vi "Review Modules Dialog.vi"(8 "error in":errorcluster, 11 "Potting Procedure in":refnum<class "Potting Procedure.lvclass">) -> (0 "error out":errorcluster, 2 "Canceled":bool, 3 "Potting Procedure out":refnum<class "Potting Procedure.lvclass">)   [LabVIEW 2017]
uses:
  Shared Components/Vec3d Class/Vec3d Class.lvclass
  Shared Components/Utils/Type Definitions/Fiducial with Source.ctl
  <vilib>/vision/Image Controls.llb/IMAQ Image.ctl
  Shared Components/Utils/Type Definitions/Physical Image.ctl
  Shared Components/Utils/Type Definitions/Multi-Fiducial Image.ctl
  Shared Components/Utils/Type Definitions/Fiducial Image.ctl
  Procedure Classes/Potting Procedure/Type Definitions/Inspect Modules.ctl
  Procedure Classes/Potting Procedure/Type Definitions/Review Modules.ctl
  Procedure Classes/Potting Procedure/Type Definitions/Inspect Modules - Module.ctl
  Procedure Classes/Potting Procedure/Potting Procedure.lvclass
panel:
  out "Current Module":cluster{"Chuck":i32, "Slot":i32}={"Chuck"=1, "Slot"=1}
  out "idx_label":string="1/10"
  in  "idx":i32
  in  "Previous":bool
  in  "Next":bool
  in  "Tab Control":T1(tab)
  in  "HDI ROC 0":bool
  in  "HDI ROC 9":bool
  in  "HDI ROC 10":bool
  in  "HDI ROC 11":bool
  in  "HDI ROC 12":bool
  in  "HDI ROC 13":bool
  in  "HDI ROC 14":bool
  in  "HDI ROC 15":bool
  in  "HDI ROC 8":bool
  in  "HDI ROC 6":bool
  in  "HDI ROC 5":bool
  in  "HDI ROC 4":bool
  in  "HDI ROC 3":bool
  in  "HDI ROC 2":bool
  in  "HDI ROC 1":bool
  out "HDI BR":T2(plugin-control)
  out "HDI BL":T2(plugin-control)
  out "HDI TR":T2(plugin-control)
  out "HDI TL":T2(plugin-control)
  in  "HDI ROC 7":bool
  in  "BBM ROC 0":bool
  in  "BBM ROC 9":bool
  in  "BBM ROC 10":bool
  in  "BBM ROC 11":bool
  in  "BBM ROC 12":bool
  in  "BBM ROC 13":bool
  in  "BBM ROC 14":bool
  in  "BBM ROC 15":bool
  in  "BBM ROC 8":bool
  in  "BBM ROC 6":bool
  in  "BBM ROC 5":bool
  in  "BBM ROC 4":bool
  in  "BBM ROC 3":bool
  in  "BBM ROC 2":bool
  in  "BBM ROC 1":bool
  in  "BBM ROC 7":bool
  out "BBM TL":T2(plugin-control)
  out "BBM TR":T2(plugin-control)
  out "BBM BL":T2(plugin-control)
  out "BBM BR":T2(plugin-control)
  in  "TBM Inner Bottom":bool
  in  "TBM Outer Bottom":bool
  in  "TBM Outer Top":bool
  in  "TBM Outer Right":bool
  in  "TBM Outer Left":bool
  in  "TBM Inner Right":bool
  in  "TBM Inner Left":bool
  in  "TBM Inner Top":bool
  out "TBM-HDI":T2(plugin-control)
  out "TBM-TBM":T2(plugin-control)
  in  "High Voltage Sensor":bool
  in  "High Voltage HDI":bool
  in  "Address Pads Upper":bool
  in  "Address Pads Lower":bool
  out "addr":T2(plugin-control) caption="Address Pads"
  out "HV-HDI":T2(plugin-control)
  out "HV-BBM":T2(plugin-control)
  in  "OK Button":bool
  in  "Cancel Button":bool
  # "Click on images to correct reference positions.\nAll error fiducials must be corrected before continuing."
  # "Pattern Recognition"
  # "Error"
  # "User Defined"
  # "Default"
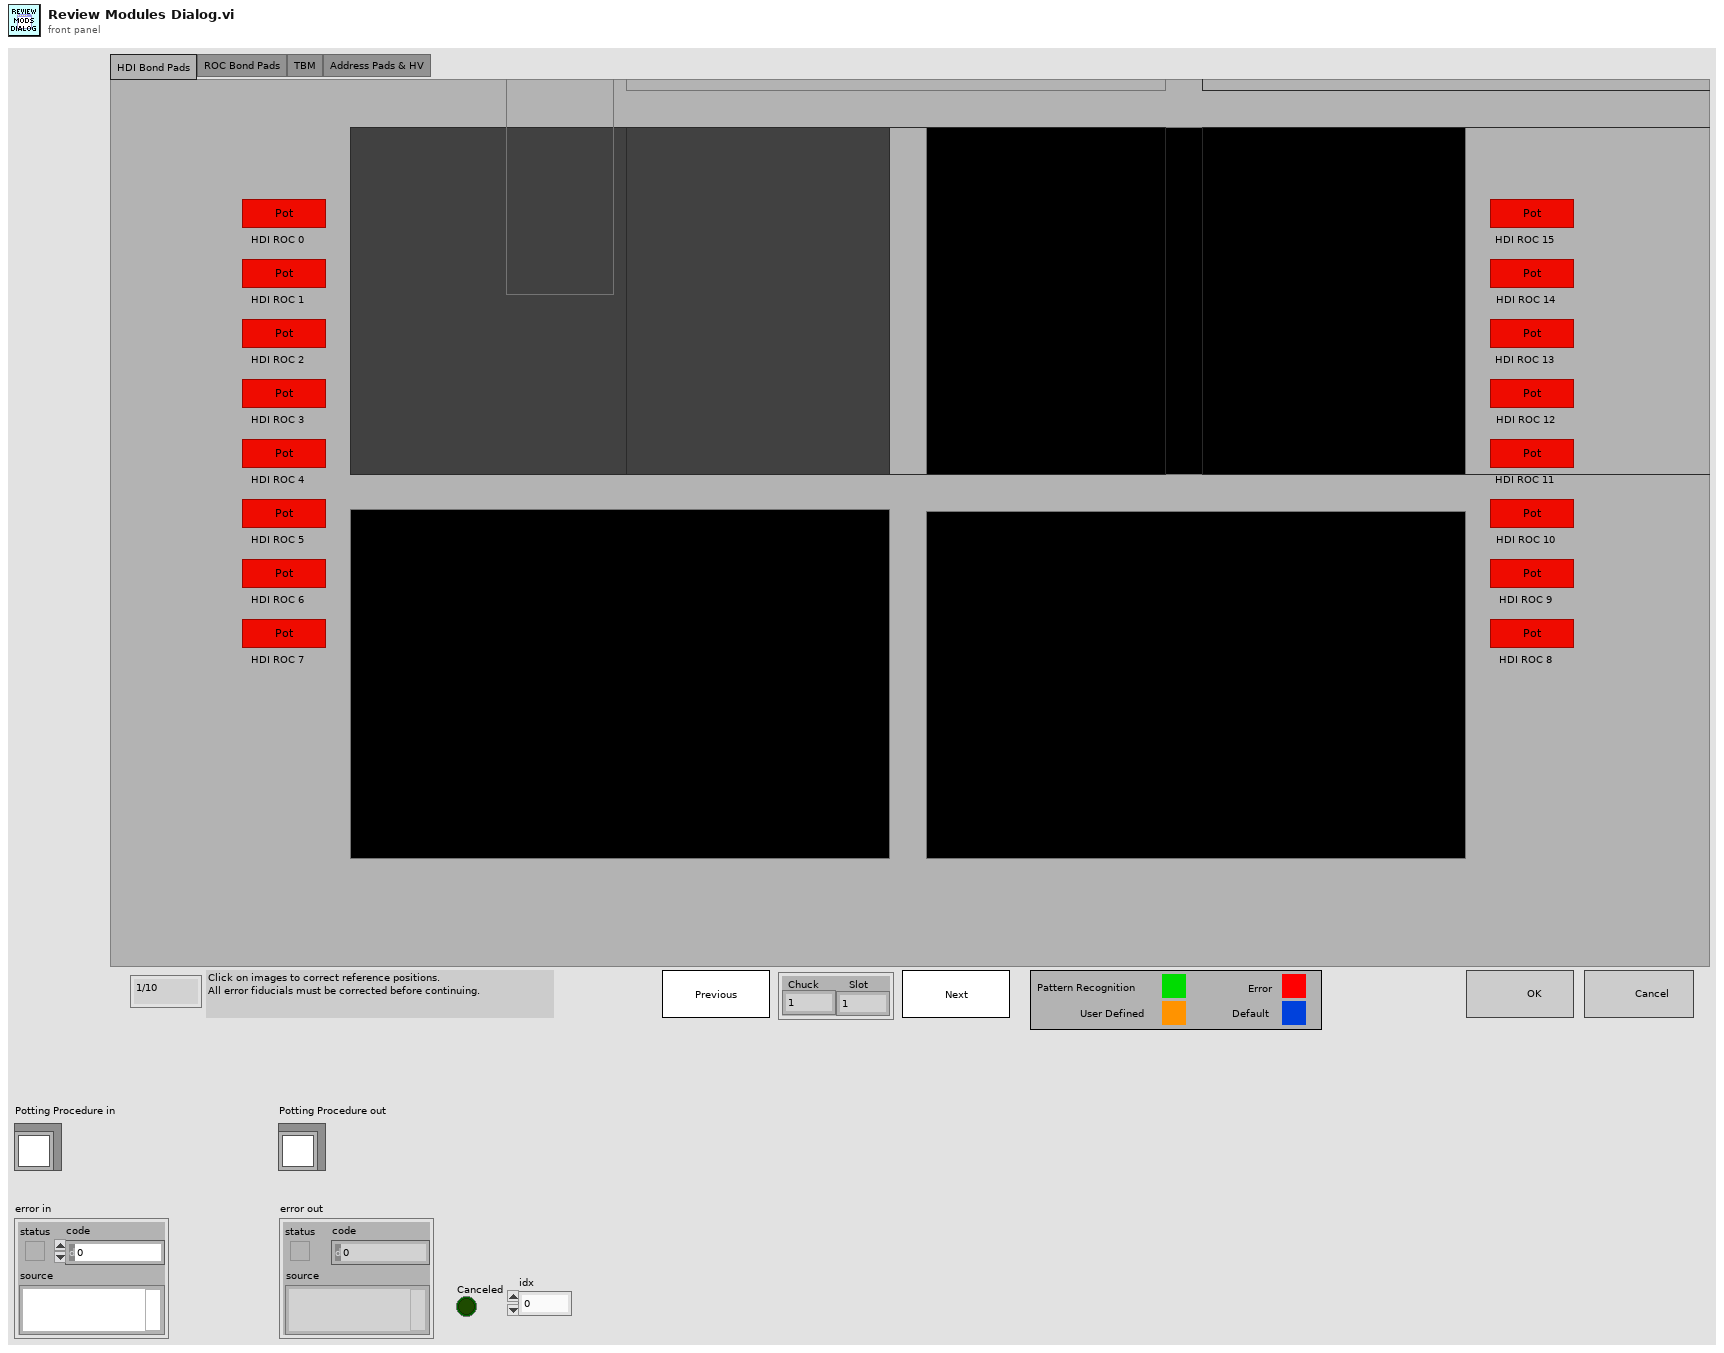
[diagram p1: front panel]
types:
  T1 = enum32{"HDI Bond Pads", "ROC Bond Pads", "TBM", "Address Pads & HV"}
  T2 = typedef "IMAQ Image.ctl" = refnum<image>
  T3 = cluster{"HDI Bond Pads":refnum<vi>[], "BBM Bond Pads":refnum<vi>[], "TBM Inner":refnum<vi>[], "TBM Outer":refnum<vi>[], "High Voltage":refnum<vi>[], "Address Pads":refnum<vi>[]}
  T4 = typedef "Inspect Modules.ctl" = cluster{"Has Been Run?":bool, "Module Positions":T5[]}
  T5 = typedef "Inspect Modules - Module.ctl" = cluster{"TBM-TBM":T6, "TBM-HDI":T6, "Address Pads":T6, "HDI Bond Pad References":T9[], "BBM Bond Pad References":T9[], "HV-HDI":T9, "HV-BBM":T9, "Chuck":i32, "Slot":i32, "Potting Selection":cluster{"HDI Bond Pads":bool[], "BBM Bond Pads":bool[], "TBM Inner":cluster{"Top":bool, "Left":bool, "Bottom":bool, "Right":bool}, "TBM Outer":cluster{"Top":bool, "Left":bool, "Bottom":bool, "Right":bool}, "Address Pads":cluster{"Top":bool, "Bottom":bool}, "High Voltage":cluster{"HDI":bool, "BBM":bool}}}
  T6 = typedef "Multi-Fiducial Image.ctl" = cluster{"Fiducial Image":T7, "Fiducials":cluster{"Selected Fiducial":T8, "fiducial name":string}[]}
  T7 = typedef "Physical Image.ctl" = cluster{"Image Position":refnum<class "Vec3d Class.lvclass">, "Image Reference":T2, "Field of View":cluster{"x(mm)":dbl, "y(mm)":dbl}}
  T8 = typedef "Fiducial with Source.ctl" = cluster{"Fiducial Image Coordinate":refnum<class "Vec3d Class.lvclass">, "Fiducial Source":enum16{"Pattern Recognition", "User", "Error", "Default"}}
  T9 = typedef "Fiducial Image.ctl" = cluster{"Fiducial Image":T7, "Selected Fiducial":T8, "fiducial name":string}
  T10 = enum16{"Pattern Recognition", "User", "Error", "Default"}
  T11 = cluster{"Top":bool, "Left":bool, "Bottom":bool, "Right":bool}
  T12 = typedef "LVPoint32TypeDef.ctl" = cluster{"Horizontal":i32, "Vertical":i32}
  T13 = cluster{"Selected Fiducial":T8, "fiducial name":string}[]
  T14 = cluster{"Selected Fiducial":T8, "fiducial name":string}
  T15 = cluster{"HDI Bond Pads":bool[], "BBM Bond Pads":bool[], "TBM Inner":cluster{"Top":bool, "Left":bool, "Bottom":bool, "Right":bool}, "TBM Outer":cluster{"Top":bool, "Left":bool, "Bottom":bool, "Right":bool}, "Address Pads":cluster{"Top":bool, "Bottom":bool}, "High Voltage":cluster{"HDI":bool, "BBM":bool}}
  T16 = typedef "eventvkey.ctl" = enum16{"ASCII", "Enter", "Return", "Shift", "Ctrl", "Alt", "Cmd", "Opt", "Caps", "NumLock", "Clear", "Break", "Up", "Down", "Left", "Right", "Insert", "Delete", "Home", "End", "PageUp", "PageDown", "Escape", "Help", "Pause", "ScrollLock", "F1", "F2", "F3", "F4", "F5", "F6", "F7", "F8", "F9", "F10", "F11", "F12", "F13", "F14", "F15", "F16", "F17", "F18", "F19", "F20", "F21", "F22", "F23", "F24", "Play", "VolumeUp", "VolumeDown", "Mute", "Two Byte Char"}
  T17 = typedef "Review Modules.ctl" = cluster{"Has Been Run?":bool}
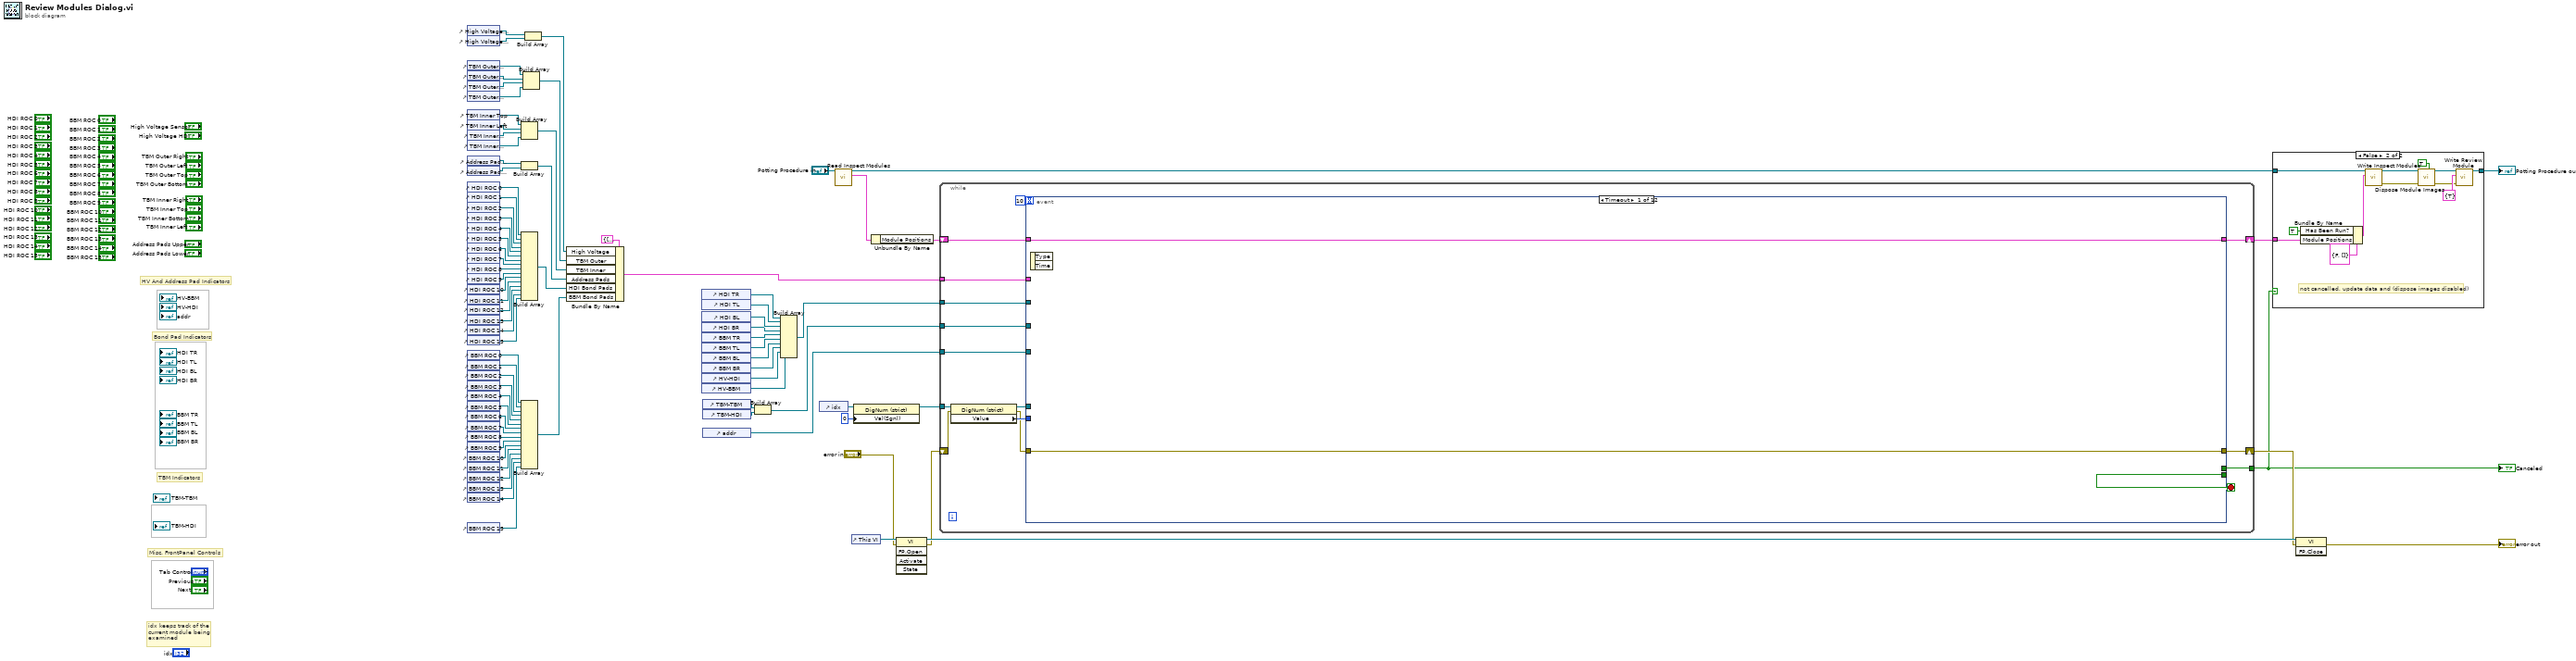
[diagram p0: block diagram]
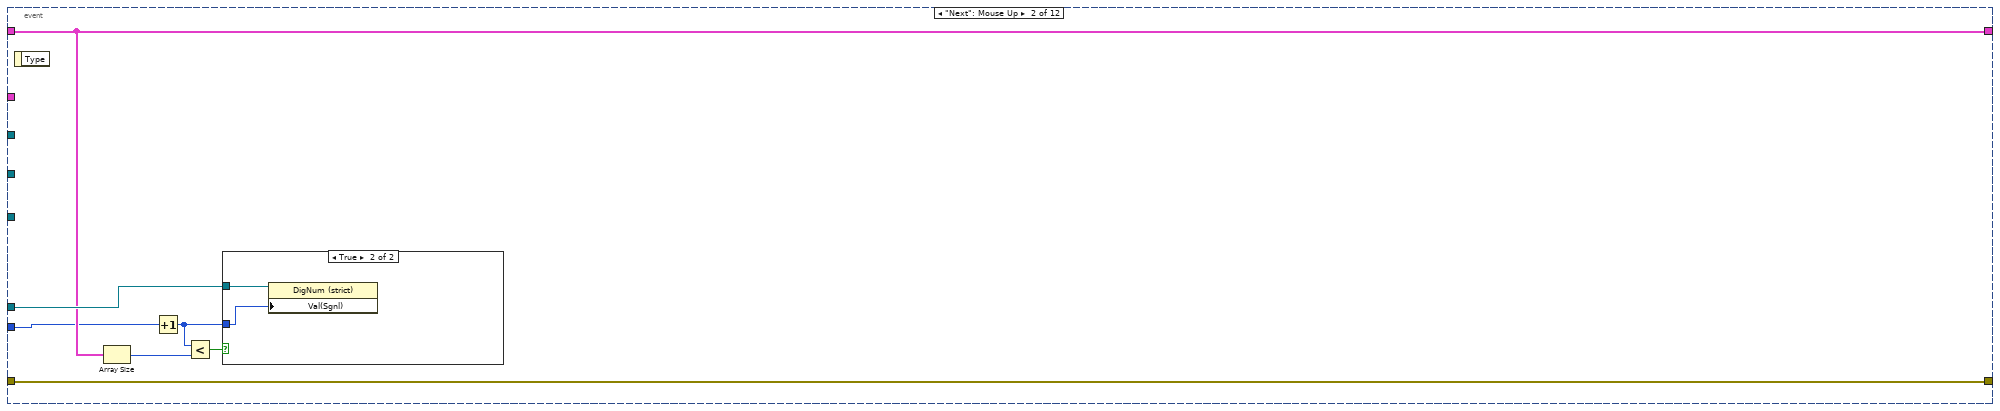
[diagram p3: hidden frame]
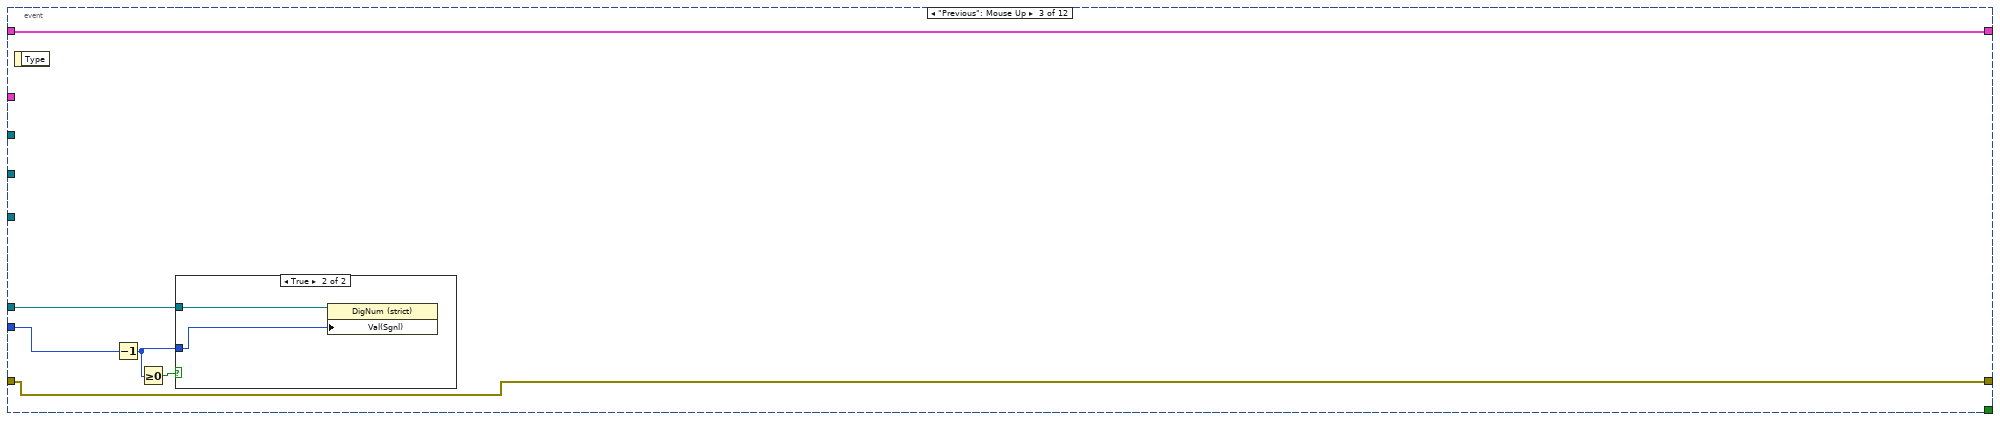
[diagram p5: hidden frame]
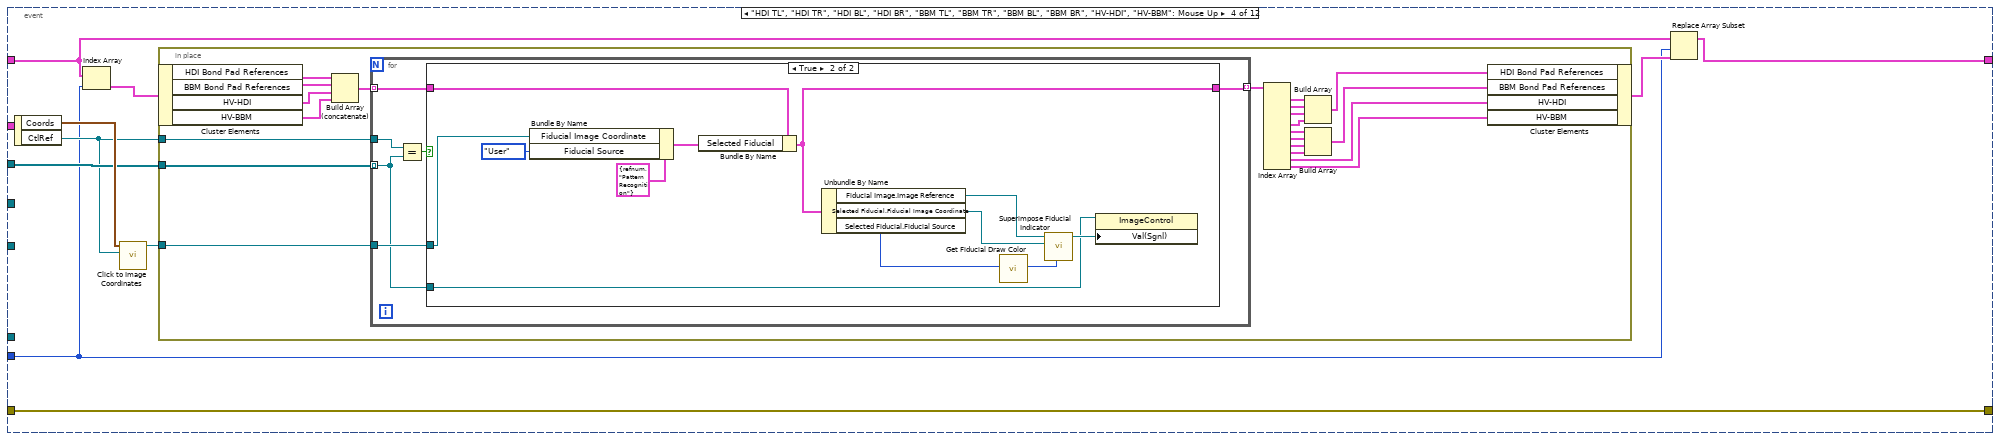
[diagram p7: hidden frame]
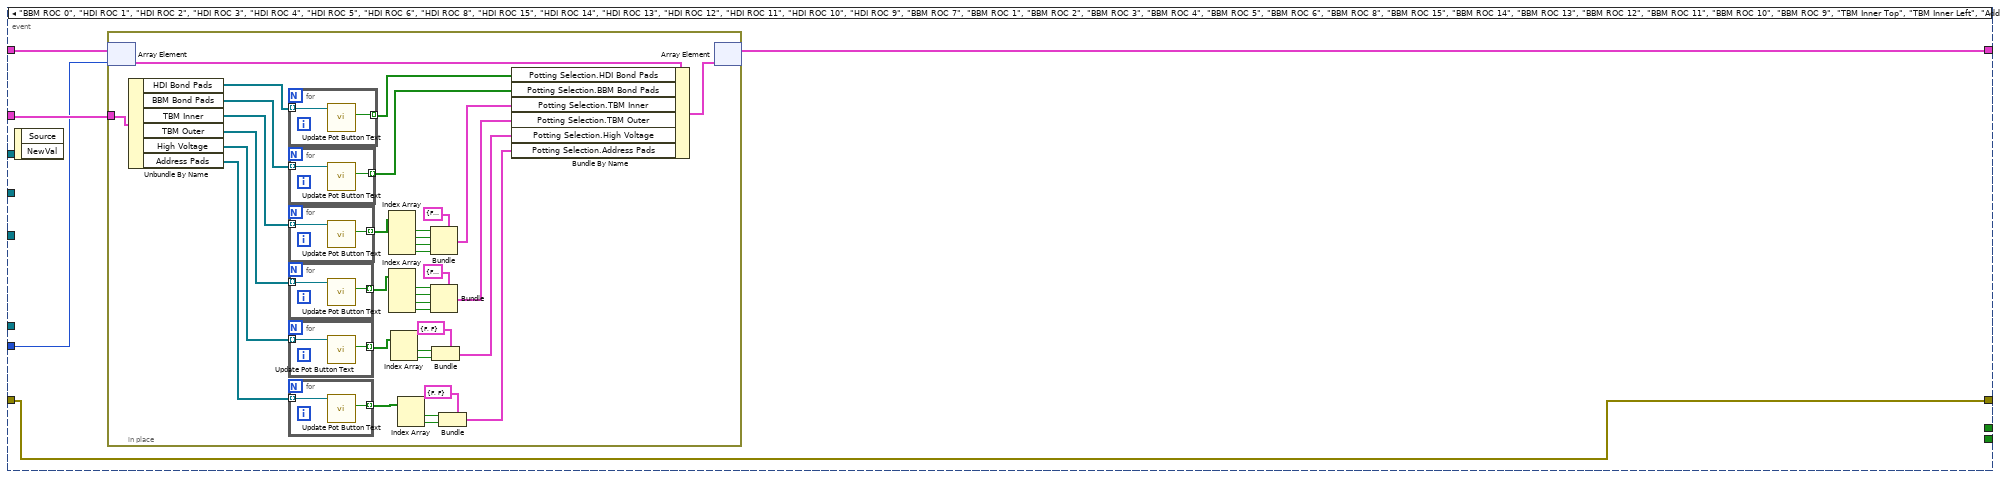
[diagram p9: hidden frame]
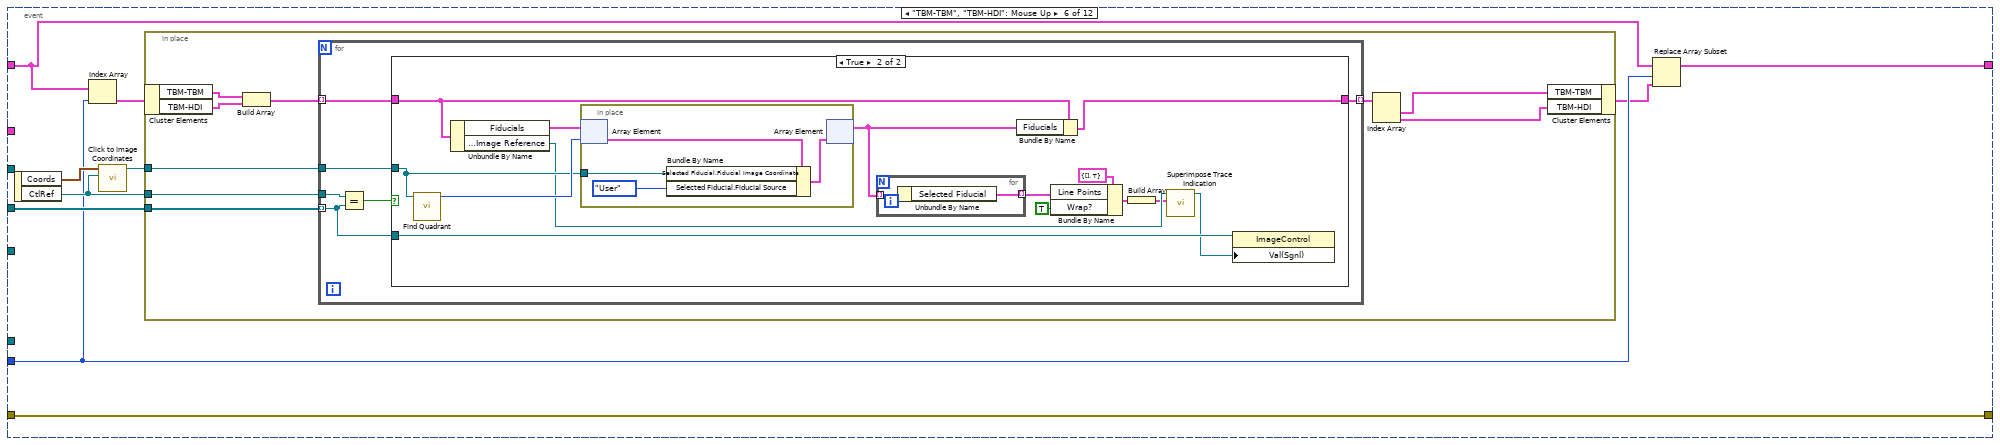
[diagram p10: hidden frame]
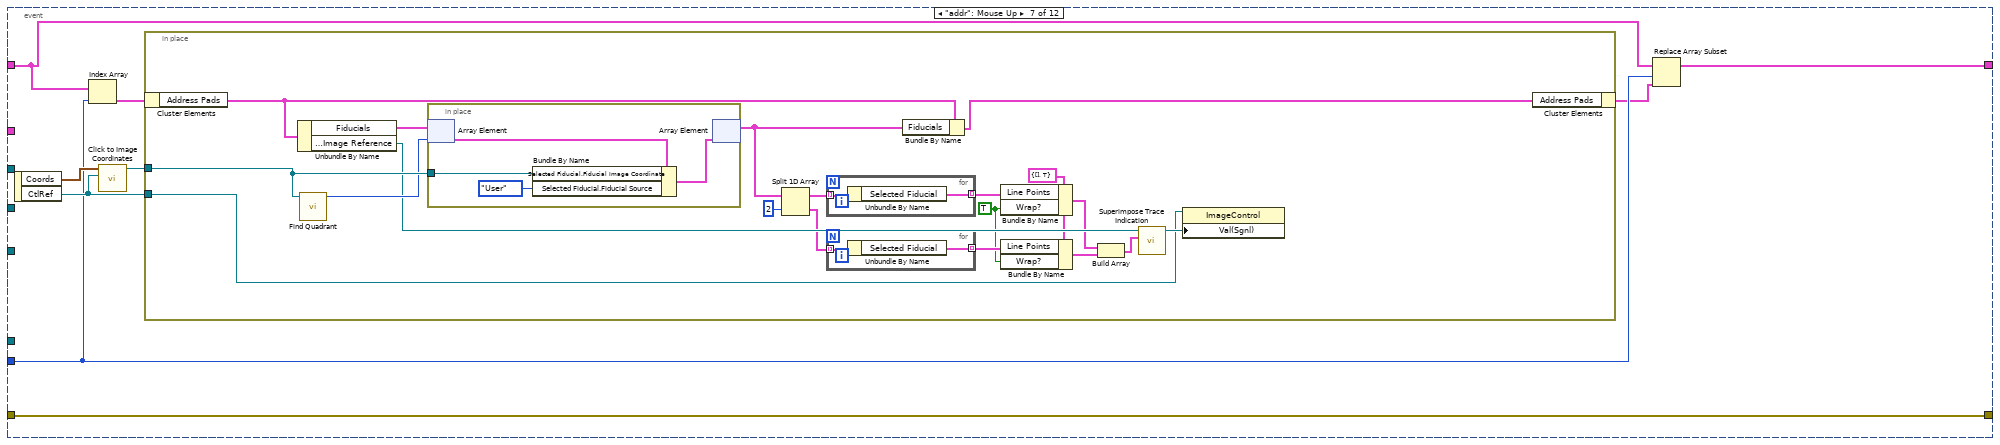
[diagram p12: hidden frame]
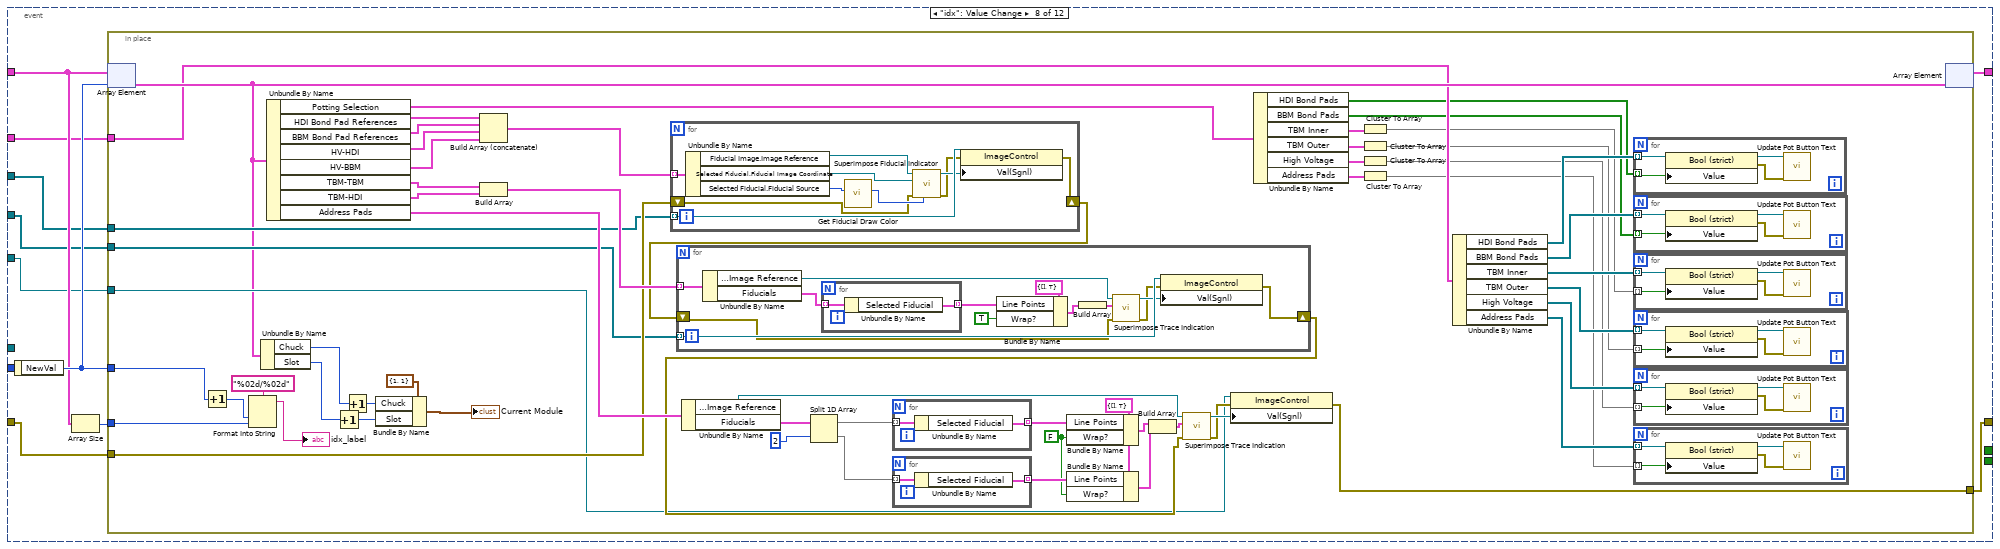
[diagram p13: hidden frame]
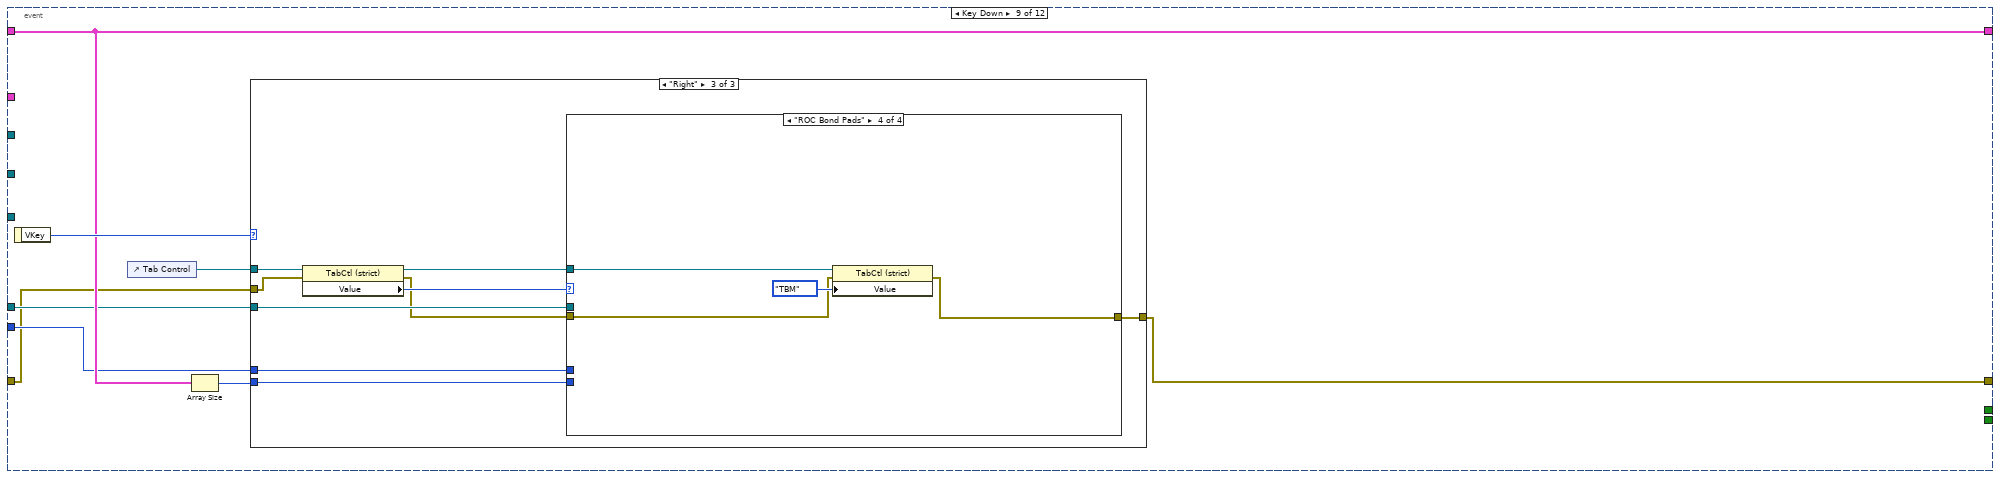
[diagram p14: hidden frame]
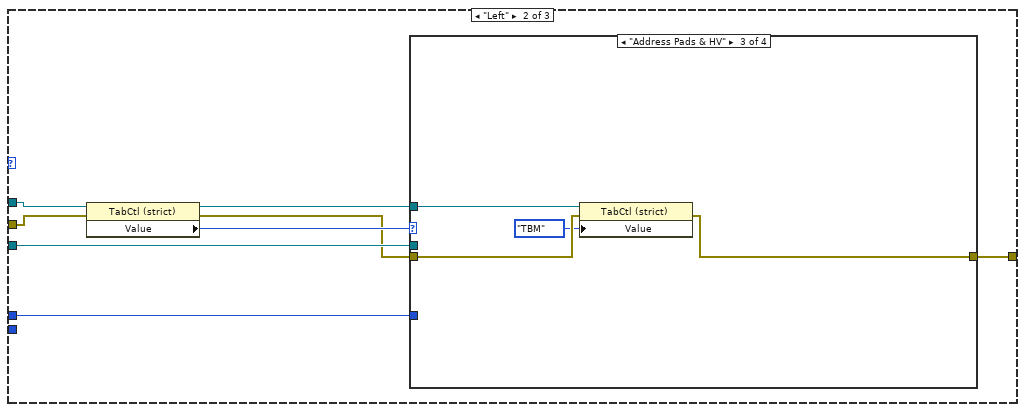
[diagram p16: hidden frame]
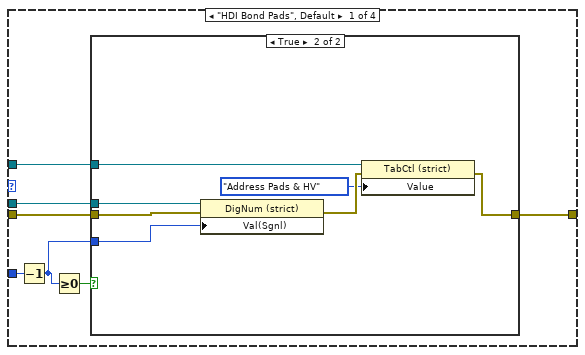
[diagram p17: hidden frame]
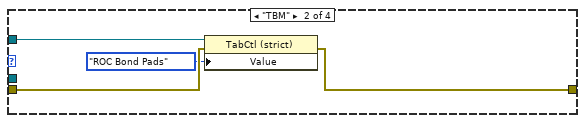
[diagram p19: hidden frame]
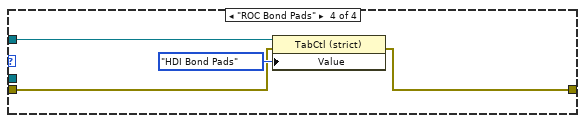
[diagram p20: hidden frame]
diagram:
  # "idx keeps track of the\ncurrent module being\nexamined"
  # "Misc. FrontPanel Controls"
  # "TBM Indicators"
  # "HV And Address Pad Indicators"
  # "Bond Pad Indicators"
  n1 = control-ref of="High Voltage HDI"() -> (w12:refnum<vi>)
  n2 = control-ref of="High Voltage Sensor"() -> (w11:refnum<vi>)
  n3 = control-ref of="TBM Outer Top"() -> (w13:refnum<vi>)
  n4 = control-ref of="TBM Outer Left"() -> (w16:refnum<vi>)
  n5 = control-ref of="TBM Outer Bottom"() -> (w15:refnum<vi>)
  n6 = control-ref of="TBM Outer Right"() -> (w14:refnum<vi>)
  n7 = control-ref of="TBM Inner Top"() -> (w17:refnum<vi>)
  n8 = control-ref of="TBM Inner Left"() -> (w19:refnum<vi>)
  n9 = control-ref of="TBM Inner Bottom"() -> (w20:refnum<vi>)
  n10 = control-ref of="TBM Inner Right"() -> (w18:refnum<vi>)
  n11 = control-ref of="Address Pads Upper"() -> (w3:refnum<vi>)
  n12 = control-ref of="Address Pads Lower"() -> (w2:refnum<vi>)
  n13 = control-ref of="HDI ROC 0"() -> (w52:refnum<vi>)
  n14 = control-ref of="HDI ROC 1"() -> (w51:refnum<vi>)
  n15 = control-ref of="HDI ROC 2"() -> (w50:refnum<vi>)
  n16 = control-ref of="HDI ROC 3"() -> (w49:refnum<vi>)
  n17 = control-ref of="HDI ROC 4"() -> (w48:refnum<vi>)
  n18 = control-ref of="HDI ROC 5"() -> (w47:refnum<vi>)
  n19 = control-ref of="HDI ROC 6"() -> (w46:refnum<vi>)
  n20 = control-ref of="HDI ROC 7"() -> (w45:refnum<vi>)
  n21 = control-ref of="HDI ROC 8"() -> (w44:refnum<vi>)
  n22 = control-ref of="HDI ROC 9"() -> (w43:refnum<vi>)
  n23 = control-ref of="HDI ROC 10"() -> (w42:refnum<vi>)
  n24 = control-ref of="HDI ROC 11"() -> (w41:refnum<vi>)
  n25 = control-ref of="HDI ROC 12"() -> (w40:refnum<vi>)
  n26 = control-ref of="HDI ROC 13"() -> (w39:refnum<vi>)
  n27 = control-ref of="HDI ROC 14"() -> (w38:refnum<vi>)
  n28 = control-ref of="HDI ROC 15"() -> (w37:refnum<vi>)
  n29 = control-ref of="BBM ROC 0"() -> (w36:refnum<vi>)
  n30 = control-ref of="BBM ROC 1"() -> (w35:refnum<vi>)
  n31 = control-ref of="BBM ROC 2"() -> (w34:refnum<vi>)
  n32 = control-ref of="BBM ROC 3"() -> (w33:refnum<vi>)
  n33 = control-ref of="BBM ROC 4"() -> (w32:refnum<vi>)
  n34 = control-ref of="BBM ROC 5"() -> (w31:refnum<vi>)
  n35 = control-ref of="BBM ROC 6"() -> (w30:refnum<vi>)
  n36 = control-ref of="BBM ROC 7"() -> (w29:refnum<vi>)
  n37 = control-ref of="BBM ROC 8"() -> (w28:refnum<vi>)
  n38 = control-ref of="BBM ROC 9"() -> (w27:refnum<vi>)
  n39 = control-ref of="BBM ROC 10"() -> (w26:refnum<vi>)
  n40 = control-ref of="BBM ROC 11"() -> (w25:refnum<vi>)
  n41 = control-ref of="BBM ROC 12"() -> (w24:refnum<vi>)
  n42 = control-ref of="BBM ROC 13"() -> (w23:refnum<vi>)
  n43 = control-ref of="BBM ROC 14"() -> (w22:refnum<vi>)
  n44 = control-ref of="BBM ROC 15"() -> (w21:refnum<vi>)
  n45 = Build Array(w17, w19, w20, w18) -> (w4:refnum<vi>[])
  n46 = Build Array(w3, w2) -> (w1:refnum<vi>[])
  n47 = Build Array(w52, w51, w50, w49, w48, w47, w46, w45, w44, w43, w42, w41, w40, w39, w38, w37) -> (w9:refnum<vi>[])
  n48 = Build Array(w36, w35, w34, w33, w32, w31, w30, w29, w28, w27, w26, w25, w24, w23, w22, w21) -> (w8:refnum<vi>[])
  n49 = Build Array(w13, w16, w15, w14) -> (w5:refnum<vi>[])
  n50 = Build Array(w12, w11) -> (w6:refnum<vi>[])
  n51 = Bundle By Name(cluster=T3 {"HDI Bond Pads"=[], "BBM Bond Pads"=[], "TBM Inner"=[], "TBM Outer"=[], "High Voltage"=[], "Address Pads"=[]}, "High Voltage"=w6, "TBM Outer"=w5, "TBM Inner"=w4, "Address Pads"=w1, "HDI Bond Pads"=w9, "BBM Bond Pads"=w8) -> (w7:T3)
  n52 = control-ref of="HDI TR"() -> (w74:refnum<vi>)
  n53 = control-ref of="HDI TL"() -> (w73:refnum<vi>)
  n54 = control-ref of="HDI BL"() -> (w72:refnum<vi>)
  n55 = control-ref of="HDI BR"() -> (w71:refnum<vi>)
  n56 = control-ref of="BBM TR"() -> (w70:refnum<vi>)
  n57 = control-ref of="BBM TL"() -> (w69:refnum<vi>)
  n58 = control-ref of="BBM BL"() -> (w68:refnum<vi>)
  n59 = control-ref of="BBM BR"() -> (w67:refnum<vi>)
  n60 = control-ref of="HV-HDI"() -> (w62:refnum<vi>)
  n61 = control-ref of="HV-BBM"() -> (w61:refnum<vi>)
  n62 = control-ref of="TBM-TBM"() -> (w65:refnum<vi>)
  n63 = control-ref of="TBM-HDI"() -> (w64:refnum<vi>)
  n64 = control-ref of="addr"() -> (w60:refnum<vi>)
  n65 = Build Array(w65, w64) -> (w63:refnum<vi>[])
  n66 = Build Array(w74, w73, w72, w71, w70, w69, w68, w67, w62, w61) -> (w66:refnum<vi>[])
  n67 = control-ref of="idx"() -> (w59:refnum<vi>)
  n68 = call-dynamic "Read Inspect Modules.vi"("Potting Procedure in"="Potting Procedure in") -> ("Inspect Modules"=w76:T4, "Potting Procedure out"=w54:refnum<class "Potting Procedure.lvclass">)  [unwired: 8 in, 1 out]
  n69 = control-ref of="This VI"() -> (w83:refnum<vi>)
  n70 = property class="DigNum (strict)"(reference=w59, "Val(Sgnl)"=0 ("Value (Signaling)")) -> (reference out=w58:refnum<vi>)  [unwired: 1 in, 1 out]
  n71 = Unbundle By Name(w76) -> ("Module Positions"=w75:T5[])
  n72 = invoke class="VI" method="FP.Open"(reference=w83, error in="error in") -> (reference out=w82:refnum<vi>, error out=w79:errorcluster)  [unwired: 3 in, 3 out]
  n73 = while {
    tunnel: [w95] -> w56
    shift-right: [w93] -> w55
    shift-left: w75 -> [w94]
    tunnel: w58 -> [w91]
    tunnel: w66 -> [w92]
    tunnel: w63 -> [w86]
    tunnel: w60 -> [w85]
    tunnel: w7 -> [w84]
    shift-right: [w96] -> w78
    shift-left: w79 -> [w88]
    stop <- w97 stop-if-true
    n74 = property class="DigNum (strict)"(reference=w91, error in=w88) -> (reference out=w90:refnum<vi>, error out=w87:errorcluster, "Value"=w89:i32)
    n75 = event shown="[0] Timeout" {
      selector: _ -> [_ _ _ _ _ _ _ _ _ _ _ _]
      dyn-events: _ -> [_ _ _ _ _ _ _ _ _ _ _ _]
      timeout: 10 -> [_ _ _ _ _ _ _ _ _ _ _ _]
      tunnel: [_ _ _ _ _ _ _ _ _ w507 w509 _] -> w97
      tunnel: [w100 w101 w110 w118 w168 w220 w266 w302 w425 w508 w511 w514] -> w96
      tunnel: w87 -> [w100 w101 w110 w118 w168 w220 w266 w307 w426 w508 w511 w514]
      tunnel: [_ _ _ _ _ _ _ _ _ w507 _ _] -> w95
      tunnel: w94 -> [w99 w103 w112 w122 w171 w222 w268 w309 w430 w506 w510 w513]
      tunnel: [w99 w103 w112 w119 w169 w221 w267 w311 w430 w506 w510 w513] -> w93
      tunnel: w90 -> [_ w105 w113 _ _ _ _ _ w427 _ _ _]
      tunnel: w92 -> [_ _ _ w125 _ _ _ w305 _ _ _ _]
      tunnel: w89 -> [_ w102 w111 w120 w170 w224 w270 _ w428 _ _ _]
      tunnel: w86 -> [_ _ _ _ _ w227 _ w304 _ _ _ _]
      tunnel: w85 -> [_ _ _ _ _ _ _ w306 _ _ _ _]
      tunnel: w84 -> [_ _ _ _ w172 _ _ w303 _ _ _ _]
      event Timeout {
        n76 = event-data() -> ()  [unwired: 1 in, 2 out]
      }
      event "Next": Mouse Up {
        n77 = event-data() -> ()  [unwired: 1 in, 1 out]
        n78 = Array Size(array=w103) -> (size(s)=w104:i32)
        n79 = Increment(x=w102) -> (x+1=w106:i32)
        n80 = Less?(x=w106, y=w104) -> (x < y?=w107:bool)
        n81 = case shown="True" w107 {
          tunnel: w106 -> [_ w108]
          tunnel: w105 -> [_ w109]
          frame False {
          }
          frame True {
            n82 = property class="DigNum (strict)"(reference=w109, "Val(Sgnl)"=w108) -> ()  [unwired: 1 in, 2 out]
          }
        }
      }
      event "Previous": Mouse Up {
        n83 = event-data() -> ()  [unwired: 1 in, 1 out]
        n84 = Decrement(x=w111) -> (x-1=w114:i32)
        n85 = Greater Or Equal To 0?(x=w114) -> (x >= 0?=w115:bool)
        n86 = case shown="True" w115 {
          tunnel: w114 -> [_ w116]
          tunnel: w113 -> [_ w117]
          frame False {
          }
          frame True {
            n87 = property class="DigNum (strict)"(reference=w117, "Val(Sgnl)"=w116) -> ()  [unwired: 1 in, 2 out]
          }
        }
      }
      event "HDI TL", "HDI TR", "HDI BL", "HDI BR", "BBM TL", "BBM TR", "BBM BL", "BBM BR", "HV-HDI", "HV-BBM": Mouse Up {
        n88 = event-data() -> ("Coords"=w127:T12, "CtlRef"=w124:refnum<vi>)  [unwired: 1 in]
        n89 = Index Array(array=w122, index=w120) -> (element=w123:T5)
        n90 = call "Click to Image Coordinates.vi"("Display Reference"=w124, "Coords"=w127) -> ("Image Coordinates"=w126:refnum<class "Vec3d Class.lvclass">)  [unwired: 8 in, 1 out]
        n91 = in-place {
          in-place-border: w126 -> [w147]
          in-place-border: w125 -> [w146]
          in-place-border: w124 -> [w145]
          n92 = in-place-cluster #1(w123) -> ("HDI Bond Pad References"=w144:T9[], "BBM Bond Pad References"=w143:T9[], "HV-HDI"=w142:T9, "HV-BBM"=w141:T9)
          n93 = Build Array (concatenate)(w144, w143, w142, w141) -> (w148:T9[])
          n94 = for {
            tunnel: w148 -> [w151] mode=indexing
            tunnel: w147 -> [w152]
            tunnel: w146 -> [w150] mode=indexing
            tunnel: w145 -> [w154]
            tunnel: [w149] -> w140 mode=indexing
            n95 = Equal?(x=w154, y=w150) -> (x = y?=w153:bool)
            n96 = case shown="True" w153 {
              tunnel: w152 -> [_ w165]
              tunnel: w151 -> [w155 w167]
              tunnel: [w155 w162] -> w149
              tunnel: w150 -> [_ w158]
              frame False {
              }
              frame True {
                n97 = Bundle By Name(cluster=T8 {"Fiducial Image Coordinate"=refnum, "Fiducial Source"=enum."Pattern Recognition"} ("Selected Fiducial"), "Fiducial Image Coordinate"=w165, "Fiducial Source"=T10."User") -> (w163:T8)
                n98 = Bundle By Name(cluster=w167, "Selected Fiducial"=w163) -> (w162:T9)
                n99 = Unbundle By Name(w162) -> ("Fiducial Image.Image Reference"=w159:T2, "Selected Fiducial.Fiducial Image Coordinate"=w160:refnum<class "Vec3d Class.lvclass">, "Selected Fiducial.Fiducial Source"=w157:T10)
                n100 = call "Get Fiducial Draw Color.vi"("Fiducial Source"=w157) -> ("Grid Line Color"=w156:u32)  [unwired: 10 in]
                n101 = call "Superimpose Fiducial Indicator.vi"("Marker Color"=w156, "Fiducial Image Coordinates"=w160, "Image In"=w159) -> ("Image Out"=w161:T2)  [unwired: 7 in, 1 out]
                n102 = property class="ImageControl"(reference=w158, "Val(Sgnl)"=w161) -> ()  [unwired: 1 in, 2 out]
              }
            }
          }
          n103 = Index Array(array=w140) -> (element #1=w139:T9, element #2=w138:T9, element #3=w137:T9, element #4=w136:T9, element #5=w134:T9, element #6=w133:T9, element #7=w132:T9, element #8=w131:T9, element #9=w129:T9, element #10=w128:T9)  [unwired: 10 in]
          n104 = Build Array(w139, w138, w137, w136) -> (w135:T9[])
          n105 = Build Array(w134, w133, w132, w131) -> (w130:T9[])
          n106 = in-place-cluster #1("HDI Bond Pad References"=w135, "BBM Bond Pad References"=w130, "HV-HDI"=w129, "HV-BBM"=w128) -> (w121:T5)
        }
        n107 = Replace Array Subset(array=w122, new element=w121, index=w120) -> (w119:T5[])
      }
      event "BBM ROC 0", "HDI ROC 1", "HDI ROC 2", "HDI ROC 3", "HDI ROC 4", "HDI ROC 5", "HDI ROC 6", "HDI ROC 8", "HDI ROC 15", "HDI ROC 14", "HDI ROC 13", "HDI ROC 12", "HDI ROC 11", "HDI ROC 10", "HDI ROC 9", "BBM ROC 7", "BBM ROC 1", "BBM ROC 2", "BBM ROC 3", "BBM ROC 4", "BBM ROC 5", "BBM ROC 6", "BBM ROC 8", "BBM ROC 15", "BBM ROC 14", "BBM ROC 13", "BBM ROC 12", "BBM ROC 11", "BBM ROC 10", "BBM ROC 9", "TBM Inner Top", "TBM Inner Left", "Address Pads Lower", "Address Pads Upper", "High Voltage HDI", "High Voltage Sensor", "TBM Inner Right", "TBM Outer Left", "TBM Outer Right", "TBM Outer Top", "TBM Outer Bottom", "TBM Inner Bottom", "HDI ROC 7", "HDI ROC 0": Value Change {
        n108 = event-data() -> ()  [unwired: 1 in, 2 out]
        n109 = in-place {
          in-place-border: w172 -> [w207]
          n110 = in-place-array #2(w171, w170) -> (w205:T5)
          n111 = Unbundle By Name(w207) -> ("HDI Bond Pads"=w206:refnum<vi>[], "BBM Bond Pads"=w203:refnum<vi>[], "TBM Inner"=w200:refnum<vi>[], "TBM Outer"=w199:refnum<vi>[], "High Voltage"=w198:refnum<vi>[], "Address Pads"=w197:refnum<vi>[])
          n112 = for {
            tunnel: w206 -> [w219] mode=indexing
            tunnel: [w218] -> w204 mode=indexing
            n113 = call "Update Pot Button Text.vi"("Button Reference"=w219) -> ("Value"=w218:bool)  [unwired: 9 in, 1 out]
          }
          n114 = for {
            tunnel: w203 -> [w217] mode=indexing
            tunnel: [w216] -> w202 mode=indexing
            n115 = call "Update Pot Button Text.vi"("Button Reference"=w217) -> ("Value"=w216:bool)  [unwired: 9 in, 1 out]
          }
          n116 = for {
            tunnel: w200 -> [w215] mode=indexing
            tunnel: [w214] -> w195 mode=indexing
            n117 = call "Update Pot Button Text.vi"("Button Reference"=w215) -> ("Value"=w214:bool)  [unwired: 9 in, 1 out]
          }
          n118 = for {
            tunnel: w199 -> [w213] mode=indexing
            tunnel: [w212] -> w184 mode=indexing
            n119 = call "Update Pot Button Text.vi"("Button Reference"=w213) -> ("Value"=w212:bool)  [unwired: 9 in, 1 out]
          }
          n120 = for {
            tunnel: w198 -> [w211] mode=indexing
            tunnel: [w210] -> w179 mode=indexing
            n121 = call "Update Pot Button Text.vi"("Button Reference"=w211) -> ("Value"=w210:bool)  [unwired: 9 in, 1 out]
          }
          n122 = for {
            tunnel: w197 -> [w209] mode=indexing
            tunnel: [w208] -> w176 mode=indexing
            n123 = call "Update Pot Button Text.vi"("Button Reference"=w209) -> ("Value"=w208:bool)  [unwired: 9 in, 1 out]
          }
          n124 = Index Array(array=w195) -> (element #1=w194:bool, element #2=w193:bool, element #3=w192:bool, element #4=w191:bool)  [unwired: 4 in]
          n125 = Index Array(array=w184) -> (element #1=w188:bool, element #2=w187:bool, element #3=w186:bool, element #4=w185:bool)  [unwired: 4 in]
          n126 = Index Array(array=w179) -> (element #1=w182:bool, element #2=w181:bool)  [unwired: 2 in]
          n127 = Index Array(array=w176) -> (element #1=w178:bool, element #2=w177:bool)  [unwired: 2 in]
          n128 = Bundle(cluster=T11 {"Top"=FALSE, "Left"=FALSE, "Bottom"=FALSE, "Right"=FALSE} ("Potting Selection.TBM Inner"), "Top"=w194, "Left"=w193, "Bottom"=w192, "Right"=w191) -> (w190:T11)
          n129 = Bundle(cluster=T11 {"Top"=FALSE, "Left"=FALSE, "Bottom"=FALSE, "Right"=FALSE} ("Potting Selection.TBM Inner"), "Top"=w188, "Left"=w187, "Bottom"=w186, "Right"=w185) -> (w183:T11)
          n130 = Bundle(cluster=cluster{"Top":bool, "Bottom":bool} {"Top"=FALSE, "Bottom"=FALSE} ("Potting Selection.Address Pads"), "Top"=w182, "Bottom"=w181) -> (w175:cluster{"Top":bool, "Bottom":bool})
          n131 = Bundle(cluster=cluster{"HDI":bool, "Sensor":bool} {"HDI"=FALSE, "Sensor"=FALSE} ("Potting Selection.High Voltage"), "HDI"=w178, "Sensor"=w177) -> (w173:cluster{"HDI":bool, "Sensor":bool})
          n132 = Bundle By Name(cluster=w205, "Potting Selection.HDI Bond Pads"=w204, "Potting Selection.BBM Bond Pads"=w202, "Potting Selection.TBM Inner"=w190, "Potting Selection.TBM Outer"=w183, "Potting Selection.High Voltage"=w175, "Potting Selection.Address Pads"=w173) -> (w201:T5)
          n133 = in-place-array #2(w201) -> (w169:T5[])  [unwired: 1 out]
        }
      }
      event "TBM-TBM", "TBM-HDI": Mouse Up {
        n134 = event-data() -> ("Coords"=w229:T12, "CtlRef"=w228:refnum<vi>)  [unwired: 1 in]
        n135 = Index Array(array=w222, index=w224) -> (element=w225:T5)
        n136 = call "Click to Image Coordinates.vi"("Display Reference"=w228, "Coords"=w229) -> ("Image Coordinates"=w226:refnum<class "Vec3d Class.lvclass">)  [unwired: 8 in, 1 out]
        n137 = in-place {
          in-place-border: w228 -> [w237]
          in-place-border: w227 -> [w236]
          in-place-border: w226 -> [w235]
          n138 = in-place-cluster #3(w225) -> ("TBM-TBM"=w234:T6, "TBM-HDI"=w233:T6)
          n139 = Build Array(w234, w233) -> (w238:T6[])
          n140 = for {
            tunnel: w238 -> [w242] mode=indexing
            tunnel: w237 -> [w244]
            tunnel: w236 -> [w240] mode=indexing
            tunnel: w235 -> [w241]
            tunnel: [w239] -> w232 mode=indexing
            n141 = Equal?(x=w244, y=w240) -> (x = y?=w243:bool)
            n142 = case shown="True" w243 {
              tunnel: w242 -> [w245 w256]
              tunnel: w241 -> [_ w257]
              tunnel: [w245 w255] -> w239
              tunnel: w240 -> [_ w247]
              frame False {
              }
              frame True {
                n143 = call "Find Quadrant.vi"("Image Coordinate"=w257) -> ("Quadrant"=w258:i32)  [unwired: 10 in]
                n144 = Unbundle By Name(w256) -> ("Fiducials"=w259:T13, "Fiducial Image.Image Reference"=w251:T2)
                n145 = in-place {
                  in-place-border: w257 -> [w263]
                  n146 = in-place-array #4(w259, w258) -> (w265:T14)
                  n147 = Bundle By Name(cluster=w265, "Selected Fiducial.Fiducial Image Coordinate"=w263, "Selected Fiducial.Fiducial Source"=T10."User") -> (w264:T14)
                  n148 = in-place-array #4(w264) -> (w254:T13)  [unwired: 1 out]
                }
                n149 = for {
                  tunnel: w254 -> [w261] mode=indexing
                  tunnel: [w260] -> w250 mode=indexing
                  n150 = Unbundle By Name(w261) -> ("Selected Fiducial"=w260:T8)
                }
                n151 = Bundle By Name(cluster=w256, "Fiducials"=w254) -> (w255:T6)
                n152 = Bundle By Name(cluster=cluster{"Line Points":T8[], "Wrap?":bool} {"Line Points"=[], "Wrap?"=TRUE} ("Line Group"), "Line Points"=w250, "Wrap?"=TRUE) -> (w253:cluster{"Line Points":T8[], "Wrap?":bool})
                n153 = Build Array(w253) -> (w248:cluster{"Line Points":T8[], "Wrap?":bool}[])
                n154 = call "Superimpose Trace Indication.vi"("Line Data"=w248, "Image In"=w251) -> ("Image Out"=w246:T2)  [unwired: 8 in, 1 out]
                n155 = property class="ImageControl"(reference=w247, "Val(Sgnl)"=w246) -> ()  [unwired: 1 in, 2 out]
              }
            }
          }
          n156 = Index Array(array=w232) -> (element #1=w231:T6, element #2=w230:T6)  [unwired: 2 in]
          n157 = in-place-cluster #3("TBM-TBM"=w231, "TBM-HDI"=w230) -> (w223:T5)
        }
        n158 = Replace Array Subset(array=w222, new element=w223, index=w224) -> (w221:T5[])
      }
      event "addr": Mouse Up {
        n159 = event-data() -> ("Coords"=w274:T12, "CtlRef"=w273:refnum<vi>)  [unwired: 1 in]
        n160 = Index Array(array=w268, index=w270) -> (element=w271:T5)
        n161 = call "Click to Image Coordinates.vi"("Display Reference"=w273, "Coords"=w274) -> ("Image Coordinates"=w272:refnum<class "Vec3d Class.lvclass">)  [unwired: 8 in, 1 out]
        n162 = in-place {
          in-place-border: w273 -> [w284]
          in-place-border: w272 -> [w293]
          w275 = cluster{"Line Points":T8[], "Wrap?":bool} {"Line Points"=[], "Wrap?"=TRUE} ("Line Group")
          w278 = TRUE ("Wrap?")
          n163 = in-place-cluster #5(w271) -> ("Address Pads"=w291:T6)
          n164 = Unbundle By Name(w291) -> ("Fiducials"=w290:T13, "Fiducial Image.Image Reference"=w288:T2)
          n165 = call "Find Quadrant.vi"("Image Coordinate"=w293) -> ("Quadrant"=w289:i32)  [unwired: 10 in]
          n166 = in-place {
            in-place-border: w293 -> [w299]
            n167 = in-place-array #6(w290, w289) -> (w301:T14)
            n168 = Bundle By Name(cluster=w301, "Selected Fiducial.Fiducial Image Coordinate"=w299, "Selected Fiducial.Fiducial Source"=T10."User") -> (w300:T14)
            n169 = in-place-array #6(w300) -> (w282:T13)  [unwired: 1 out]
          }
          n170 = Split 1D Array(array=w282, index=2) -> (first subarray=w281:T13, second subarray=w280:T13)
          n171 = for {
            tunnel: [w296] -> _ mode=indexing
            tunnel: [w297] -> w287 mode=indexing
            tunnel: w281 -> [w296] mode=indexing
            n172 = Unbundle By Name(w296) -> ("Selected Fiducial"=w297:T8)
          }
          n173 = for {
            tunnel: w280 -> [w295] mode=indexing
            tunnel: [w294] -> w283 mode=indexing
            n174 = Unbundle By Name(w295) -> ("Selected Fiducial"=w294:T8)
          }
          n175 = Bundle By Name(cluster=w291, "Fiducials"=w282) -> (w292:T6)
          n176 = Bundle By Name(cluster=w275, "Line Points"=w287, "Wrap?"=w278) -> (w277:cluster{"Line Points":T8[], "Wrap?":bool})
          n177 = Bundle By Name(cluster=w275, "Line Points"=w283, "Wrap?"=w278) -> (w276:cluster{"Line Points":T8[], "Wrap?":bool})
          n178 = Build Array(w277, w276) -> (w286:cluster{"Line Points":T8[], "Wrap?":bool}[])
          n179 = call "Superimpose Trace Indication.vi"("Line Data"=w286, "Image In"=w288) -> ("Image Out"=w285:T2)  [unwired: 8 in, 1 out]
          n180 = property class="ImageControl"(reference=w284, "Val(Sgnl)"=w285) -> ()  [unwired: 1 in, 2 out]
          n181 = in-place-cluster #5("Address Pads"=w292) -> (w269:T5)
        }
        n182 = Replace Array Subset(array=w268, new element=w269, index=w270) -> (w267:T5[])
      }
      event "idx": Value Change {
        n183 = event-data() -> ("NewVal"=w310:i32)  [unwired: 1 in]
        n184 = Array Size(array=w309) -> (size(s)=w308:i32)
        n185 = in-place {
          in-place-border: w310 -> [w331]
          in-place-border: w308 -> [w330]
          in-place-border: w307 -> [w329]
          in-place-border: w306 -> [w328]
          in-place-border: w305 -> [w327]
          in-place-border: w304 -> [w326]
          in-place-border: w303 -> [w323]
          in-place-border: [w312] -> w302
          w346 = FALSE ("Wrap?")
          w345 = cluster{"Line Points":T8[], "Wrap?":bool} {"Line Points"=[], "Wrap?"=TRUE} ("Line Group")
          n186 = in-place-array #7(w309, w310) -> (w325:T5)
          n187 = Increment(x=w331) -> (x+1=w338:i32)
          n188 = Format Into String(format string="%02d/%02d", w338, w330) -> (resulting string=→"idx_label":string)  [unwired: 2 in, 1 out]
          n189 = Unbundle By Name(w325) -> ("Chuck"=w333:i32, "Slot"=w332:i32)
          n190 = Unbundle By Name(w325) -> ("Potting Selection"=w324:T15, "HDI Bond Pad References"=w365:T9[], "BBM Bond Pad References"=w364:T9[], "HV-HDI"=w363:T9, "HV-BBM"=w362:T9, "TBM-TBM"=w361:T6, "TBM-HDI"=w360:T6, "Address Pads"=w352:T6)
          n191 = Increment(x=w332) -> (x+1=w337:i32)
          n192 = Increment(x=w333) -> (x+1=w336:i32)
          n193 = Bundle By Name(cluster=cluster{"Chuck":i32, "Slot":i32} {"Chuck"=1, "Slot"=1} ("Current Module"), "Chuck"=w336, "Slot"=w337) -> (→"Current Module":cluster{"Chuck":i32, "Slot":i32})
          n194 = Build Array (concatenate)(w365, w364, w363, w362) -> (w359:T9[])
          n195 = Build Array(w361, w360) -> (w358:T6[])
          n196 = for {
            tunnel: w327 -> [w395] mode=indexing
            tunnel: w359 -> [w400] mode=indexing
            shift-right: [w391] -> w343
            shift-left: w329 -> [w393]
            n197 = Unbundle By Name(w400) -> ("Fiducial Image.Image Reference"=w399:T2, "Selected Fiducial.Fiducial Image Coordinate"=w398:refnum<class "Vec3d Class.lvclass">, "Selected Fiducial.Fiducial Source"=w397:T10)
            n198 = call "Get Fiducial Draw Color.vi"("Fiducial Source"=w397) -> ("Grid Line Color"=w396:u32)  [unwired: 10 in]
            n199 = call "Superimpose Fiducial Indicator.vi"("Marker Color"=w396, "error in"=w393, "Fiducial Image Coordinates"=w398, "Image In"=w399) -> ("error out"=w392:errorcluster, "Image Out"=w394:T2)  [unwired: 6 in]
            n200 = property class="ImageControl"(reference=w395, error in=w392, "Val(Sgnl)"=w394) -> (error out=w391:errorcluster)  [unwired: 1 out]
          }
          n201 = for {
            tunnel: w326 -> [w386] mode=indexing
            tunnel: w358 -> [w388] mode=indexing
            shift-right: [w376] -> w342
            shift-left: w343 -> [w378]
            n202 = Unbundle By Name(w388) -> ("Fiducial Image.Image Reference"=w387:T2, "Fiducials"=w384:T13)
            n203 = for {
              tunnel: w384 -> [w390] mode=indexing
              tunnel: [w389] -> w382 mode=indexing
              n204 = Unbundle By Name(w390) -> ("Selected Fiducial"=w389:T8)
            }
            n205 = Bundle By Name(cluster=cluster{"Line Points":T8[], "Wrap?":bool} {"Line Points"=[], "Wrap?"=TRUE} ("Line Group"), "Line Points"=w382, "Wrap?"=TRUE) -> (w380:cluster{"Line Points":T8[], "Wrap?":bool})
            n206 = Build Array(w380) -> (w379:cluster{"Line Points":T8[], "Wrap?":bool}[])
            n207 = call "Superimpose Trace Indication.vi"("error in"=w378, "Line Data"=w379, "Image In"=w387) -> ("error out"=w377:errorcluster, "Image Out"=w385:T2)  [unwired: 7 in]
            n208 = property class="ImageControl"(reference=w386, error in=w377, "Val(Sgnl)"=w385) -> (error out=w376:errorcluster)  [unwired: 1 out]
          }
          n209 = Unbundle By Name(w352) -> ("Fiducial Image.Image Reference"=w357:T2, "Fiducials"=w351:T13)
          n210 = Split 1D Array(array=w351, index=2) -> (first subarray=w349:T13, second subarray=w348:T13)
          n211 = for {
            tunnel: w349 -> [w375] mode=indexing
            tunnel: [w374] -> w355 mode=indexing
            n212 = Unbundle By Name(w375) -> ("Selected Fiducial"=w374:T8)
          }
          n213 = for {
            tunnel: w348 -> [w373] mode=indexing
            tunnel: [w372] -> w347 mode=indexing
            n214 = Unbundle By Name(w373) -> ("Selected Fiducial"=w372:T8)
          }
          n215 = Bundle By Name(cluster=w345, "Line Points"=w355, "Wrap?"=w346) -> (w354:cluster{"Line Points":T8[], "Wrap?":bool})
          n216 = Bundle By Name(cluster=w345, "Line Points"=w347, "Wrap?"=w346) -> (w344:cluster{"Line Points":T8[], "Wrap?":bool})
          n217 = Build Array(w354, w344) -> (w353:cluster{"Line Points":T8[], "Wrap?":bool}[])
          n218 = call "Superimpose Trace Indication.vi"("error in"=w342, "Line Data"=w353, "Image In"=w357) -> ("error out"=w341:errorcluster, "Image Out"=w356:T2)  [unwired: 7 in]
          n219 = property class="ImageControl"(reference=w328, error in=w341, "Val(Sgnl)"=w356) -> (error out=w312:errorcluster)  [unwired: 1 out]
          n220 = Unbundle By Name(w324) -> ("HDI Bond Pads"=w322:bool[], "BBM Bond Pads"=w321:bool[], "TBM Inner"=w320:T11, "TBM Outer"=w318:T11, "High Voltage"=w317:cluster{"HDI":bool, "BBM":bool}, "Address Pads"=w316:cluster{"Top":bool, "Bottom":bool})
          n221 = Cluster To Array(cluster=w320) -> (array=w319:bool[])
          n222 = Cluster To Array(cluster=w318) -> (array=w315:bool[])
          n223 = Cluster To Array(cluster=w317) -> (array=w314:bool[])
          n224 = Cluster To Array(cluster=w316) -> (array=w313:bool[])
          n225 = Unbundle By Name(w323) -> ("HDI Bond Pads"=w371:refnum<vi>[], "BBM Bond Pads"=w370:refnum<vi>[], "TBM Inner"=w369:refnum<vi>[], "TBM Outer"=w368:refnum<vi>[], "High Voltage"=w367:refnum<vi>[], "Address Pads"=w366:refnum<vi>[])
          n226 = for {
            tunnel: w371 -> [w422] mode=indexing
            tunnel: w322 -> [w424] mode=indexing
            n227 = property class="Bool (strict)"(reference=w422, "Value"=w424) -> (reference out=w421:refnum<vi>, error out=w423:errorcluster)  [unwired: 1 in]
            n228 = call "Update Pot Button Text.vi"("error in"=w423, "Button Reference"=w421) -> ()  [unwired: 8 in, 2 out]
          }
          n229 = for {
            tunnel: w370 -> [w420] mode=indexing
            tunnel: w321 -> [w419] mode=indexing
            n230 = property class="Bool (strict)"(reference=w420, "Value"=w419) -> (reference out=w417:refnum<vi>, error out=w418:errorcluster)  [unwired: 1 in]
            n231 = call "Update Pot Button Text.vi"("error in"=w418, "Button Reference"=w417) -> ()  [unwired: 8 in, 2 out]
          }
          n232 = for {
            tunnel: w369 -> [w416] mode=indexing
            tunnel: w319 -> [w415] mode=indexing
            n233 = property class="Bool (strict)"(reference=w416, "Value"=w415) -> (reference out=w413:refnum<vi>, error out=w414:errorcluster)  [unwired: 1 in]
            n234 = call "Update Pot Button Text.vi"("error in"=w414, "Button Reference"=w413) -> ()  [unwired: 8 in, 2 out]
          }
          n235 = for {
            tunnel: w368 -> [w412] mode=indexing
            tunnel: w315 -> [w411] mode=indexing
            n236 = property class="Bool (strict)"(reference=w412, "Value"=w411) -> (reference out=w409:refnum<vi>, error out=w410:errorcluster)  [unwired: 1 in]
            n237 = call "Update Pot Button Text.vi"("error in"=w410, "Button Reference"=w409) -> ()  [unwired: 8 in, 2 out]
          }
          n238 = for {
            tunnel: w367 -> [w408] mode=indexing
            tunnel: w314 -> [w407] mode=indexing
            n239 = property class="Bool (strict)"(reference=w408, "Value"=w407) -> (reference out=w405:refnum<vi>, error out=w406:errorcluster)  [unwired: 1 in]
            n240 = call "Update Pot Button Text.vi"("error in"=w406, "Button Reference"=w405) -> ()  [unwired: 8 in, 2 out]
          }
          n241 = for {
            tunnel: w366 -> [w404] mode=indexing
            tunnel: w313 -> [w403] mode=indexing
            n242 = property class="Bool (strict)"(reference=w404, "Value"=w403) -> (reference out=w401:refnum<vi>, error out=w402:errorcluster)  [unwired: 1 in]
            n243 = call "Update Pot Button Text.vi"("error in"=w402, "Button Reference"=w401) -> ()  [unwired: 8 in, 2 out]
          }
          n244 = in-place-array #7(w325) -> (w311:T5[])  [unwired: 1 out]
        }
      }
      event Key Down {
        n245 = event-data() -> ("VKey"=w432:T16)  [unwired: 1 in]
        n246 = control-ref of="Tab Control"() -> (w431:refnum<vi>)
        n247 = Array Size(array=w430) -> (size(s)=w429:i32)
        n248 = case shown="\"Right\"" w432 {
          tunnel: w431 -> [_ w437 w477]
          tunnel: w429 -> [_ _ w473]
          tunnel: w428 -> [_ w438 w472]
          tunnel: w427 -> [_ w439 w474]
          tunnel: w426 -> [w433 w436 w471]
          tunnel: [w433 w434 w469] -> w425
          frame "ASCII", Default {
          }
          frame "Left" {
            n249 = property class="TabCtl (strict)"(reference=w437, error in=w436) -> (reference out=w440:refnum<vi>, error out=w435:errorcluster, "Value"=w441:T1)
            n250 = case shown="\"Address Pads & HV\"" w441 {
              tunnel: w440 -> [w448 w460 w464 w467]
              tunnel: w439 -> [w447 _ _ _]
              tunnel: w438 -> [w446 _ _ _]
              tunnel: w435 -> [w443 w459 w463 w466]
              tunnel: [w442 w458 w462 w465] -> w434
              frame "HDI Bond Pads", Default {
                n251 = Decrement(x=w446) -> (x-1=w444:i32)
                n252 = Greater Or Equal To 0?(x=w444) -> (x >= 0?=w445:bool)
                n253 = case shown="True" w445 {
                  tunnel: w447 -> [_ w456]
                  tunnel: w448 -> [_ w455]
                  tunnel: w444 -> [_ w454]
                  tunnel: w443 -> [w449 w453]
                  tunnel: [w449 w451] -> w442
                  frame False {
                  }
                  frame True {
                    n254 = property class="DigNum (strict)"(reference=w456, error in=w453, "Val(Sgnl)"=w454) -> (error out=w452:errorcluster)  [unwired: 1 out]
                    n255 = property class="TabCtl (strict)"(reference=w455, error in=w452, "Value"=T1."Address Pads & HV") -> (error out=w451:errorcluster)  [unwired: 1 out]
                  }
                }
              }
              frame "TBM" {
                n256 = property class="TabCtl (strict)"(reference=w460, error in=w459, "Value"=T1."ROC Bond Pads") -> (error out=w458:errorcluster)  [unwired: 1 out]
              }
              frame "Address Pads & HV" {
                n257 = property class="TabCtl (strict)"(reference=w464, error in=w463, "Value"=T1."TBM") -> (error out=w462:errorcluster)  [unwired: 1 out]
              }
              frame "ROC Bond Pads" {
                n258 = property class="TabCtl (strict)"(reference=w467, error in=w466, "Value"=T1."HDI Bond Pads") -> (error out=w465:errorcluster)  [unwired: 1 out]
              }
            }
          }
          frame "Right" {
            n259 = property class="TabCtl (strict)"(reference=w477, error in=w471) -> (reference out=w475:refnum<vi>, error out=w470:errorcluster, "Value"=w476:T1)
            n260 = case shown="\"ROC Bond Pads\"" w476 {
              tunnel: w475 -> [w481 w485 w488 w504]
              tunnel: w474 -> [_ _ w490 _]
              tunnel: w473 -> [_ _ w492 _]
              tunnel: w472 -> [_ _ w493 _]
              tunnel: w470 -> [w480 w484 w487 w503]
              tunnel: [w479 w483 w486 w502] -> w469
              frame "HDI Bond Pads", Default {
                n261 = property class="TabCtl (strict)"(reference=w481, error in=w480, "Value"=T1."ROC Bond Pads") -> (error out=w479:errorcluster)  [unwired: 1 out]
              }
              frame "TBM" {
                n262 = property class="TabCtl (strict)"(reference=w485, error in=w484, "Value"=T1."Address Pads & HV") -> (error out=w483:errorcluster)  [unwired: 1 out]
              }
              frame "Address Pads & HV" {
                n263 = Increment(x=w493) -> (x+1=w489:i32)
                n264 = Less?(x=w489, y=w492) -> (x < y?=w491:bool)
                n265 = case shown="True" w491 {
                  tunnel: w490 -> [_ w501]
                  tunnel: w489 -> [_ w500]
                  tunnel: w488 -> [_ w499]
                  tunnel: w487 -> [w494 w498]
                  tunnel: [w494 w496] -> w486
                  frame False {
                  }
                  frame True {
                    n266 = property class="DigNum (strict)"(reference=w501, error in=w498, "Val(Sgnl)"=w500) -> (error out=w497:errorcluster)  [unwired: 1 out]
                    n267 = property class="TabCtl (strict)"(reference=w499, error in=w497, "Value"=T1."HDI Bond Pads") -> (error out=w496:errorcluster)  [unwired: 1 out]
                  }
                }
              }
              frame "ROC Bond Pads" {
                n268 = property class="TabCtl (strict)"(reference=w504, error in=w503, "Value"=T1."TBM") -> (error out=w502:errorcluster)  [unwired: 1 out]
              }
            }
          }
        }
      }
      event "Cancel Button": Mouse Up {
        w507 = TRUE
        n269 = event-data() -> ()  [unwired: 1 in, 2 out]
      }
      event "OK Button": Mouse Up {
        # "Check that there are no\nError Fiducials"
        n270 = event-data() -> ()  [unwired: 1 in, 2 out]
        n271 = call "Verify Module Positions.vi"("Module Positions In"=w510) -> ("All Good"=w509:bool)  [unwired: 9 in, 1 out]
        n272 = case shown="False" w509 {
          frame False {
            n273 = One Button Dialog(message="Cannot Proceed with any \"Error\" markers.\nCorrect these before proceeding") -> ()  [unwired: 1 in, 1 out]
          }
          frame True {
          }
        }
      }
      event Panel Close? {
        # "This event disables the windows \"X\""
        n274 = event-data() -> ()  [unwired: 1 in, 3 out]
        n275 = event-data("Discard?"=FALSE) -> ()  [unwired: 1 in, 1 out]
      }
    }
  }
  "Canceled" <- w56
  n276 = case shown="False" w56 {
    tunnel: w55 -> [_ w526]
    tunnel: w54 -> [w516 w528]
    tunnel: [w516 w522] -> w53
    frame True {
      # "cancelled, do nothing"
    }
    frame False {
      # "not cancelled, update data and (dispose images disabled)"
      n277 = Bundle By Name(cluster=T4 {"Has Been Run?"=FALSE, "Module Positions"=[]} ("Inspect Modules"), "Has Been Run?"=TRUE, "Module Positions"=w526) -> (w524:T4)
      n278 = call-dynamic "Write Inspect Modules.vi"("Inspect Modules"=w524, "Potting Procedure in"=w528) -> ("error out"=w519:errorcluster, "Potting Procedure out"=w521:refnum<class "Potting Procedure.lvclass">)  [unwired: 8 in]
      n279 = call-dynamic "Dispose Module Images.vi"("Archive"=TRUE, "error in"=w519, "Potting Procedure in"=w521) -> ("error out"=w518:errorcluster, "Potting Procedure out"=w520:refnum<class "Potting Procedure.lvclass">)  [unwired: 7 in]
      n280 = call-dynamic "Write Review Module.vi"("error in (no error)"=w518, "Review Modules"=T17 {"Has Been Run?"=TRUE}, "Potting Procedure in"=w520) -> ("Potting Procedure out"=w522:refnum<class "Potting Procedure.lvclass">)  [unwired: 7 in, 1 out]
    }
  }
  "Potting Procedure out" <- w53
  n281 = invoke class="VI" method="FP.Close"(reference=w82, error in=w78) -> (error out=→"error out":errorcluster)  [unwired: 1 in, 2 out]
